vi "Boiler Controller.vi"(8 "error in":errorcluster, 9 "Controller Configuration":T1, 10 "Notifiers":T2, 11 "Message Queues":T3) -> (0 "error out":errorcluster)   [LabVIEW 2014, in "Controller.lvlib"]
uses:
  Controller.lvlib
  support/Message Queue/All Message Queues.ctl
  support/Message Queue/Message Cluster.ctl
  support/Notifiers/Notifiers.ctl
  Controller Configuration.ctl
  controls/MHL UI Data.ctl
  controls/MHL Status.ctl
  support/Boiler System Globals.vi
  <vilib>/Utility/error.llb/Error Cluster From Error Code.vi
  <vilib>/ErrorRing/Error Ring.xnode
  support/Message Queue/Message Queue.lvlib
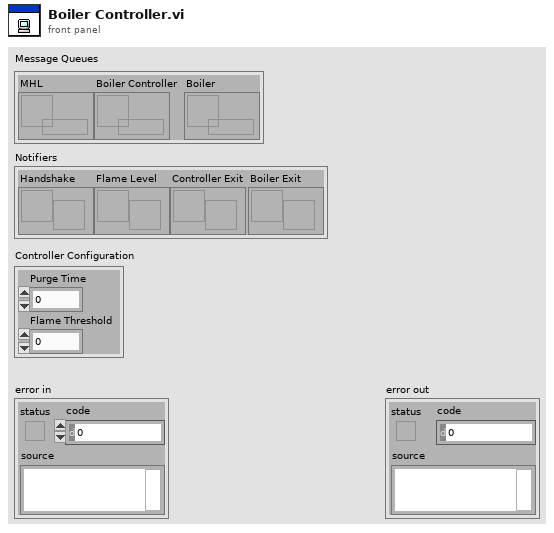
[diagram p1: front panel]
types:
  T1 = typedef "Controller.lvlib/Controller Configuration.ctl" = cluster{"Purge Time":u32, "Flame Threshold":u32}
  T2 = typedef "Notifiers.ctl" = cluster{"Handshake":refnum<notifier>, "Flame Level":refnum<notifier>, "Controller Exit":refnum<notifier>, "Boiler Exit":refnum<notifier>}
  T3 = typedef "Message Queue.lvlib/All Message Queues.ctl" = cluster{"MHL":refnum<queue>, "Boiler Controller":refnum<queue>, "Boiler":refnum<queue>}
  T4 = enum16{"open", "replace", "create", "open or create", "replace or create", "replace or create with confirmation"}
  T5 = typedef "MHL Status.ctl" = enum16{"Lockout", "Ready", "Pre-Purge", "Pre-Purge Complete", "Pilot On", "Boiler Running", "Shutdown", "Purge"}
  T6 = typedef "MHL UI Data.ctl" = cluster{"Status":string, "Fuel Control Valve":u32, "Primary Fan":bool, "Pilot Gas Valve":bool, "Pilot":bool, "Forced Draft Fan":bool, "MHL Status":T5}
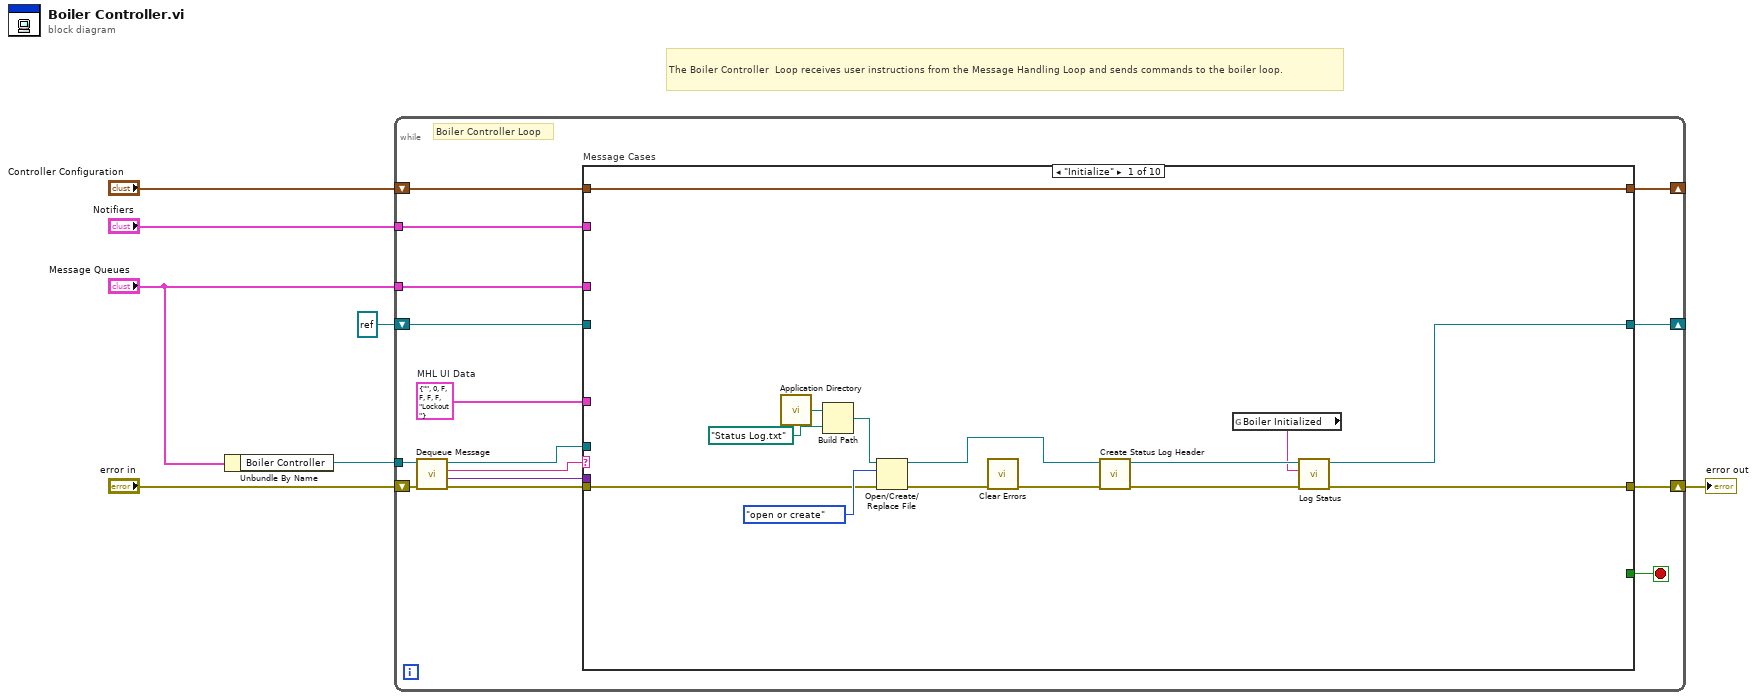
[diagram p0: block diagram]
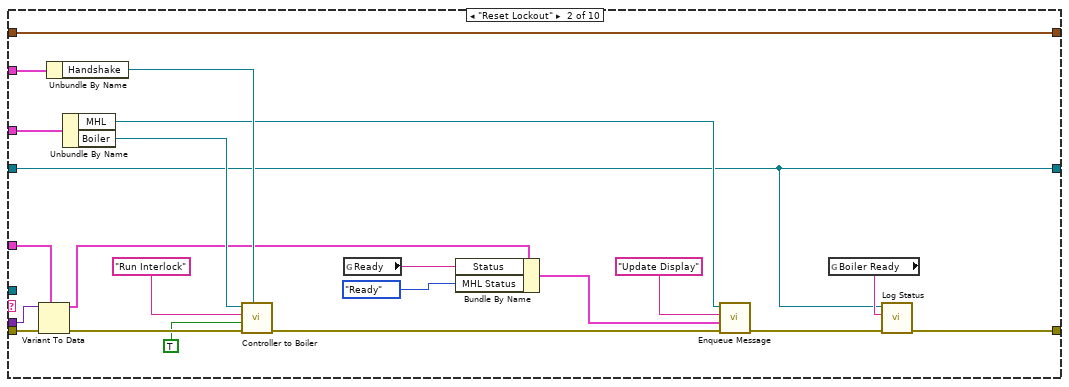
[diagram p2: hidden frame]
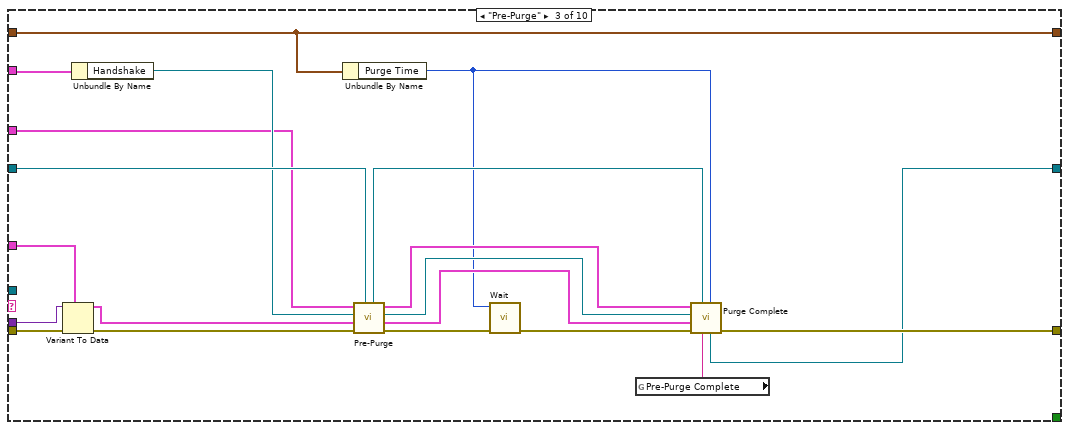
[diagram p3: hidden frame]
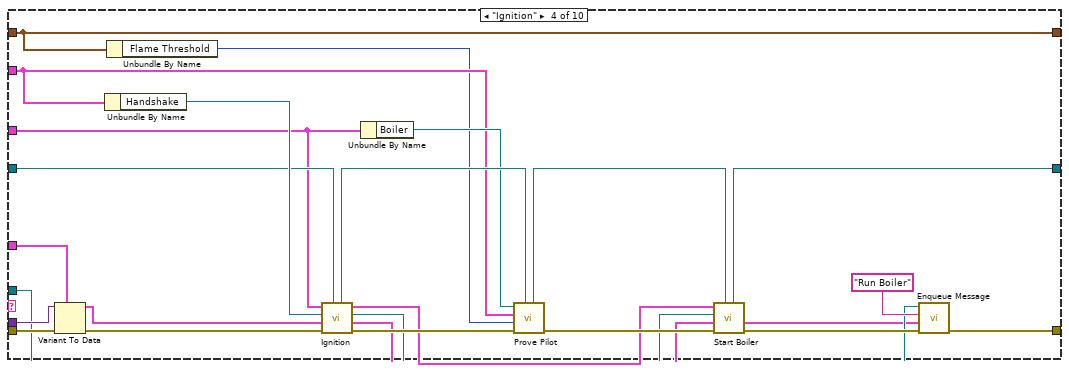
[diagram p4: hidden frame]
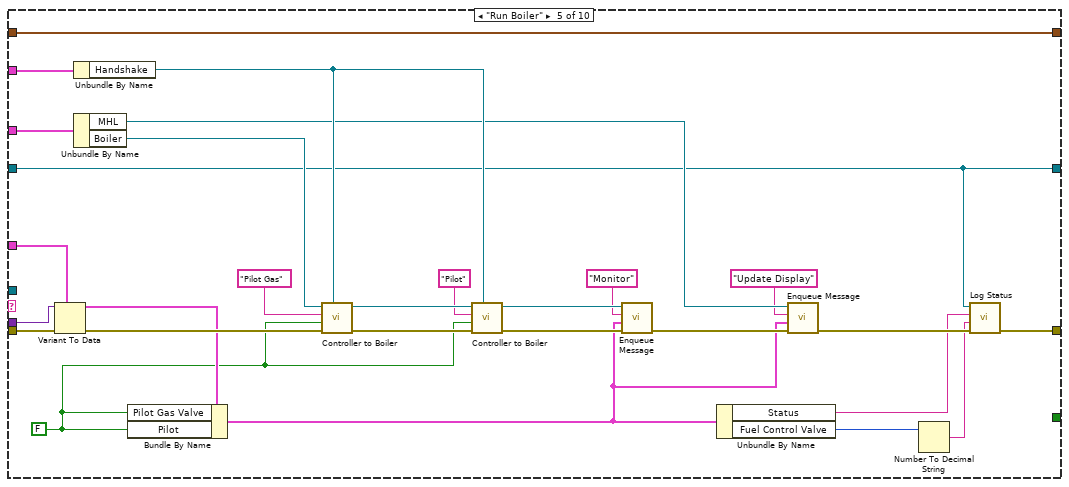
[diagram p5: hidden frame]
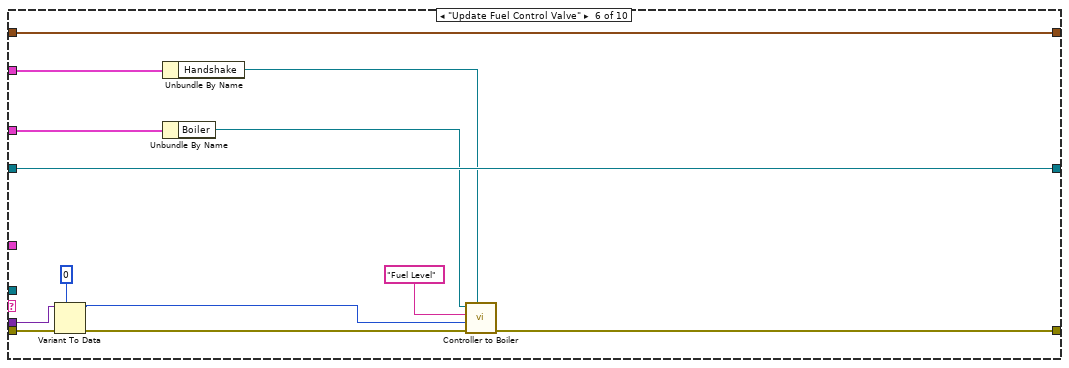
[diagram p6: hidden frame]
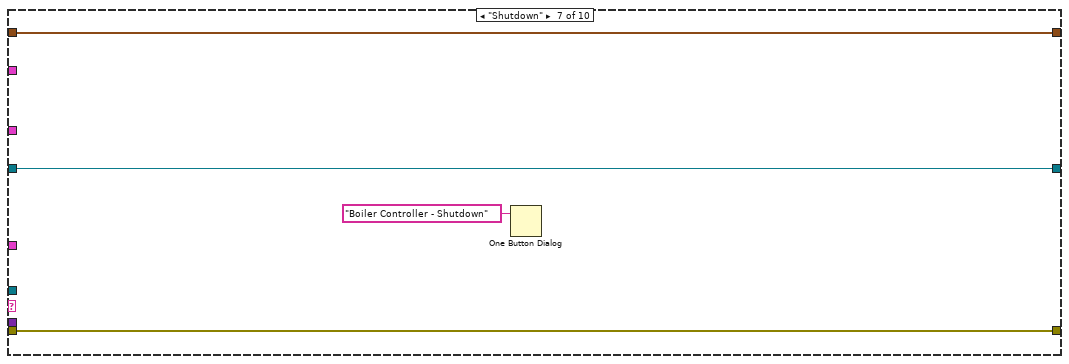
[diagram p7: hidden frame]
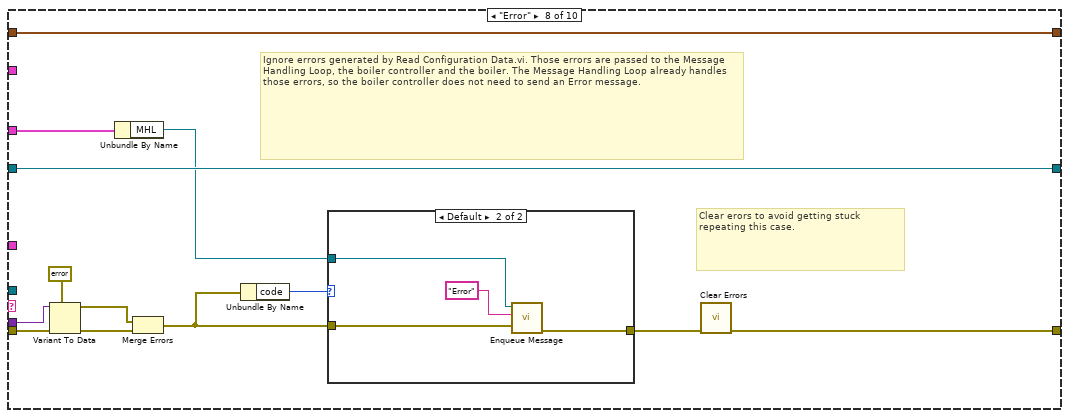
[diagram p8: hidden frame]
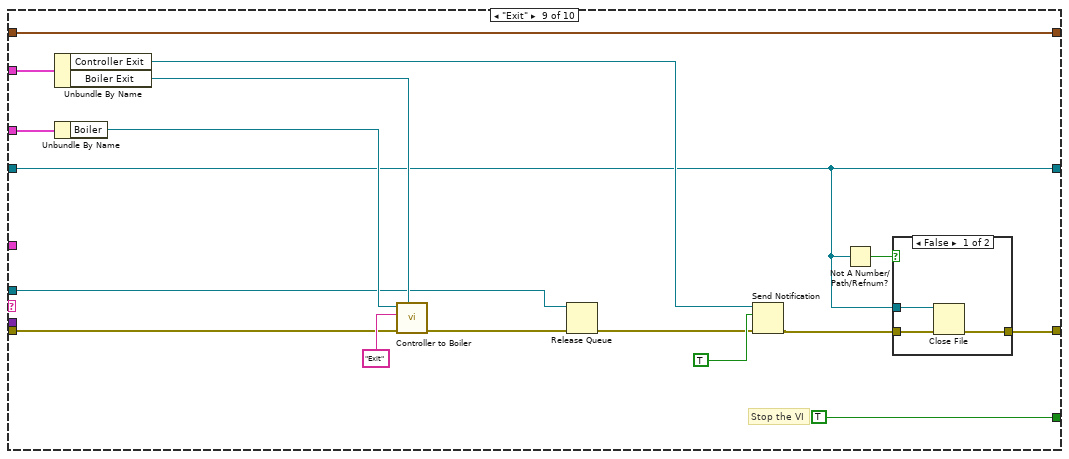
[diagram p10: hidden frame]
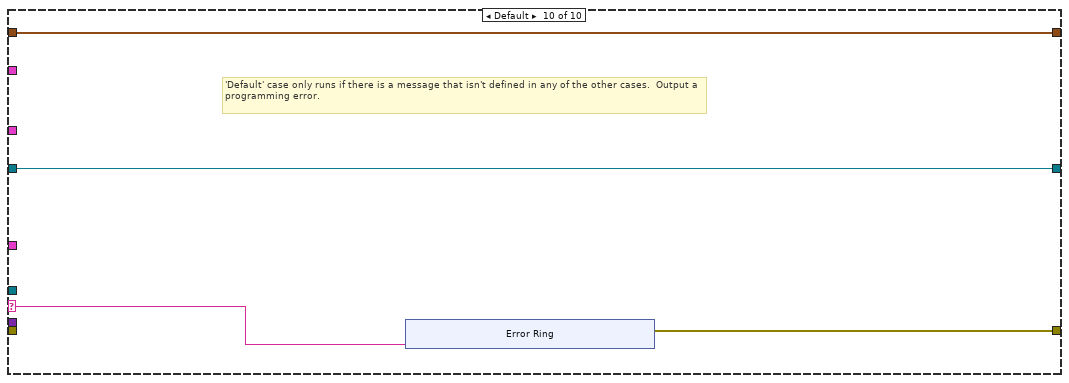
[diagram p12: hidden frame]
diagram:
  # "The Boiler Controller  Loop receives user instructions from the Message Handling Loop and sends commands to the boiler loop."
  n1 = Unbundle By Name("Message Queues") -> ("Boiler Controller"=w5:refnum<queue>)
  n2 = while {
    tunnel: w5 -> [w16]
    shift-right: [w15] -> w7
    shift-left: "error in" -> [w21]
    tunnel: "Message Queues" -> [w14]
    tunnel: "Notifiers" -> [w13]
    shift-right: [w12] -> _
    shift-left: refnum<file> refnum ("Log File Refnum out") -> [w11]
    shift-right: [w8] -> _
    shift-left: "Controller Configuration" -> [w9]
    stop <- w22 stop-if-true
    w10 = T6 {"Status"="", "Fuel Control Valve"=0, "Primary Fan"=FALSE, "Pilot Gas Valve"=FALSE, "Pilot"=FALSE, "Forced Draft Fan"=FALSE, "MHL Status"=enum."Lockout"}  # MHL UI Data
    # "Boiler Controller Loop"
    n3 = call "Dequeue Message.vi"("error in (no error)"=w21, "Message Queue"=w16) -> ("error out"=w20:errorcluster, "Message Data"=w18:variant, "Message"=w19:string, "dup Message Queue"=w17:refnum<queue>)  [unwired: 6 in]
    n4 = case "Message Cases" shown="\"Initialize\"" w19 {
      selector: w19 -> [_ _ _ _ _ _ _ _ _ w190]
      tunnel: w17 -> [_ _ _ w91 _ _ _ _ w176 _]
      tunnel: w20 -> [w26 w58 w78 w103 w131 w144 w148 w160 w175 _]
      tunnel: [w27 w54 w66 w98 w127 w140 w148 w151 w168 w191] -> w15
      tunnel: [_ _ _ _ _ _ _ _ TRUE _] -> w22
      tunnel: w18 -> [_ w53 w76 w97 w126 w139 _ w158 _ _]
      tunnel: w14 -> [_ w51 w70 w88 w122 w136 _ w161 w173 _]
      tunnel: w13 -> [_ w49 w73 w86 w121 w135 _ _ w172 _]
      tunnel: [w25 w39 w64 w79 w108 w143 w146 w155 w167 w189] -> w12
      tunnel: w11 -> [_ w39 w72 w93 w108 w143 w146 w155 w167 w189]
      tunnel: w10 -> [_ w52 w75 w96 w115 _ _ _ _ _]
      tunnel: w9 -> [w24 w37 w68 w85 w130 w142 w145 w154 w171 w188]
      tunnel: [w24 w37 w68 w85 w130 w142 w145 w154 w171 w188] -> w8
      frame "Initialize" {
        n5 = call <vilib>:"Application Directory.vi"() -> ("Application Directory"=w29:path)
        n6 = Build Path(base path=w29, name or relative path=path "Status Log.txt") -> (appended path=w33:path)
        n7 = Open/Create/Replace File(file path (use dialog)=w33, error in=w26, operation (0:open)=T4."open or create") -> (refnum out=w30:refnum<file>, error out=w31:errorcluster)  [unwired: 3 in, 1 out]
        n8 = call <vilib>:"Clear Errors.vi"("error in (no error)"=w31) -> ("error out"=w23:errorcluster)  [unwired: 5 in, 1 out]
        n9 = call "Create Status Log Header.vi"("error in"=w23, "Log File Refnum in"=w30) -> ("error out"=w36:errorcluster, "Log File Refnum out"=w35:refnum<file>)  [unwired: 8 in]
        n10 = global read "Boiler System Globals.vi" "Boiler Initialized"() -> (w34:string)
        n11 = call "Log Status.vi"("error in"=w36, "Event String"=w34, "Log File Refnum In"=w35) -> ("error out"=w27:errorcluster, "Log File Refnum Out"=w25:refnum<file>)  [unwired: 7 in]
      }
      frame "Reset Lockout" {
        n12 = Variant To Data(error in=w58, type=w52, Variant=w53) -> (data=w45:T6, error out=w57:errorcluster)
        n13 = Unbundle By Name(w49) -> ("Handshake"=w48:refnum<notifier>)
        n14 = Unbundle By Name(w51) -> ("MHL"=w41:refnum<queue>, "Boiler"=w50:refnum<queue>)
        n15 = call "Controller to Boiler.vi"("Notifier"=w48, "error in"=w57, "Message Data"=TRUE, "Message"="Run Interlock", "Boiler Queue in"=w50) -> ("error out"=w56:errorcluster)  [unwired: 4 in, 2 out]
        n16 = global read "Boiler System Globals.vi" "Ready"() -> (w44:string)
        n17 = Bundle By Name(cluster=w45, "Status"=w44, "MHL Status"=MHL_Status."Ready") -> (w43:T6)
        n18 = call "Enqueue Message.vi"("error in (no error)"=w56, "Message Data"=w43, "Message"="Update Display", "Message Queue"=w41) -> ("error out"=w55:errorcluster)  [unwired: 6 in, 1 out]
        n19 = global read "Boiler System Globals.vi" "Boiler Ready"() -> (w40:string)
        n20 = call "Log Status.vi"("error in"=w55, "Event String"=w40, "Log File Refnum In"=w39) -> ("error out"=w54:errorcluster)  [unwired: 7 in, 1 out]
      }
      frame "Pre-Purge" {
        n21 = Variant To Data(error in=w78, type=w75, Variant=w76) -> (data=w74:T6, error out=w77:errorcluster)
        n22 = Unbundle By Name(w73) -> ("Handshake"=w71:refnum<notifier>)
        n23 = Unbundle By Name(w68) -> ("Purge Time"=w60:u32)
        n24 = call "Pre-Purge.vi"("Log File Refnum in"=w72, "error in"=w77, "UI Data in"=w74, "Handshake Notifier in"=w71, "Message Queues in"=w70) -> ("error out"=w69:errorcluster, "UI Data out"=w63:T6, "Handshake Notifier out"=w62:refnum<notifier>, "Message Queues out"=w61:T3, "Log File Refnum out"=w65:refnum<file>)  [unwired: 2 in]
        n25 = call "Wait.vi"("error in"=w69, "Purge Time (s)"=w60) -> ("error out"=w67:errorcluster)  [unwired: 9 in]
        n26 = global read "Boiler System Globals.vi" "Pre-Purge Complete"() -> (w59:string)
        n27 = call "Purge Complete.vi"("Purge Time"=w60, "Status"=w59, "Log File Refnum in"=w65, "error in"=w67, "UI Data in"=w63, "Handshake Notifier in"=w62, "Message Queues in"=w61) -> ("error out"=w66:errorcluster, "Log File Refnum out"=w64:refnum<file>)  [unwired: 3 out]
      }
      frame "Ignition" {
        n28 = Variant To Data(error in=w103, type=w96, Variant=w97) -> (data=w95:T6, error out=w102:errorcluster)
        n29 = Unbundle By Name(w86) -> ("Handshake"=w94:refnum<notifier>)
        n30 = Unbundle By Name(w85) -> ("Flame Threshold"=w84:u32)
        n31 = call "Ignition.vi"("Log File Refnum in"=w93, "error in"=w102, "UI Data in"=w95, "Handshake Notifier in"=w94, "Message Queues in"=w88) -> ("error out"=w101:errorcluster, "UI Data out"=w83:T6, "Handshake Notifier out"=w82:refnum<notifier>, "Message Queues out"=w81:T3, "Log File Refnum out"=w89:refnum<file>)  [unwired: 2 in]
        n32 = Unbundle By Name(w88) -> ("Boiler"=w87:refnum<queue>)
        n33 = call "Prove Pilot.vi"("Log File Refnum in"=w89, "error in"=w101, "Flame Threshold"=w84, "Notifiers in"=w86, "Boiler Queue in"=w87) -> ("error out"=w100:errorcluster, "Log File Refnum out"=w80:refnum<file>)  [unwired: 3 in, 2 out]
        n34 = call "Start Boiler.vi"("Log File Refnum in"=w80, "error in"=w100, "UI Data in"=w83, "Handshake Notifier in"=w82, "Message Queues in"=w81) -> ("error out"=w99:errorcluster, "UI Data out"=w90:T6, "Log File Refnum out"=w79:refnum<file>)  [unwired: 2 in, 2 out]
        n35 = call "Enqueue Message.vi"("error in (no error)"=w99, "Message Data"=w90, "Message"="Run Boiler", "Message Queue"=w91) -> ("error out"=w98:errorcluster)  [unwired: 6 in, 1 out]
      }
      frame "Run Boiler" {
        w111 = FALSE ("Pilot Gas Valve")
        n36 = Variant To Data(error in=w131, type=w115, Variant=w126) -> (data=w114:T6, error out=w129:errorcluster)
        n37 = Unbundle By Name(w121) -> ("Handshake"=w120:refnum<notifier>)
        n38 = Unbundle By Name(w122) -> ("MHL"=w116:refnum<queue>, "Boiler"=w119:refnum<queue>)
        n39 = Bundle By Name(cluster=w114, "Pilot Gas Valve"=w111, "Pilot"=w111) -> (w107:T6)
        n40 = call "Controller to Boiler.vi"("Notifier"=w120, "error in"=w129, "Message Data"=w111, "Message"="Pilot Gas", "Boiler Queue in"=w119) -> ("error out"=w125:errorcluster, "Queue out"=w118:refnum<queue>)  [unwired: 4 in, 1 out]
        n41 = call "Controller to Boiler.vi"("Notifier"=w120, "error in"=w125, "Message Data"=w111, "Message"="Pilot", "Boiler Queue in"=w118) -> ("error out"=w124:errorcluster, "Queue out"=w117:refnum<queue>)  [unwired: 4 in, 1 out]
        n42 = call "Enqueue Message.vi"("error in (no error)"=w124, "Message Data"=w107, "Message"="Monitor", "Message Queue"=w117) -> ("error out"=w123:errorcluster)  [unwired: 6 in, 1 out]
        n43 = Unbundle By Name(w107) -> ("Status"=w104:string, "Fuel Control Valve"=w106:u32)
        n44 = call "Enqueue Message.vi"("error in (no error)"=w123, "Message Data"=w107, "Message"="Update Display", "Message Queue"=w116) -> ("error out"=w128:errorcluster)  [unwired: 6 in, 1 out]
        n45 = Number To Decimal String(number=w106) -> (decimal integer string=w105:string)  [unwired: 1 in]
        n46 = call "Log Status.vi"("error in"=w128, "Event Data String (-)"=w105, "Event String"=w104, "Log File Refnum In"=w108) -> ("error out"=w127:errorcluster)  [unwired: 6 in, 1 out]
      }
      frame "Update Fuel Control Valve" {
        n47 = Variant To Data(error in=w144, type=u32 0, Variant=w139) -> (data=w133:u32, error out=w141:errorcluster)
        n48 = Unbundle By Name(w135) -> ("Handshake"=w134:refnum<notifier>)
        n49 = Unbundle By Name(w136) -> ("Boiler"=w137:refnum<queue>)
        n50 = call "Controller to Boiler.vi"("Notifier"=w134, "error in"=w141, "Message Data"=w133, "Message"="Fuel Level", "Boiler Queue in"=w137) -> ("error out"=w140:errorcluster)  [unwired: 4 in, 2 out]
      }
      frame "Shutdown" {
        n51 = One Button Dialog(message="Boiler Controller - Shutdown") -> ()  [unwired: 1 in, 1 out]
      }
      frame "Error" {
        # "Ignore errors generated by Read Configuration Data.vi. Those errors are passed to the Message Handling Loop, the boiler controller and the boiler. The Message Handling Loop already handles those errors, so the boiler controller does not need to send an Error message."
        # "Clear erors to avoid getting stuck repeating this case."
        n52 = Variant To Data(error in=w160, type=errorcluster {"status"=FALSE, "code"=0, "source"=""} ("error out"), Variant=w158) -> (data=w156:errorcluster, error out=w157:errorcluster)
        n53 = Unbundle By Name(w161) -> ("MHL"=w150:refnum<queue>)
        n54 = Merge Errors(w156, w157) -> (w149:errorcluster)
        n55 = Unbundle By Name(w149) -> ("code"=w152:i32)
        n56 = case shown="Default" w152 {
          tunnel: w150 -> [_ w165]
          tunnel: [w162 w164] -> w153
          tunnel: w149 -> [w162 w163]
          frame 5000..5002 {
          }
          frame Default {
            n57 = call "Enqueue Message.vi"("Message Data"=w163, "Message"="Error", "Message Queue"=w165) -> ("error out"=w164:errorcluster)  [unwired: 7 in, 1 out]
          }
        }
        n58 = call <vilib>:"Clear Errors.vi"("error in (no error)"=w153) -> ("error out"=w151:errorcluster)  [unwired: 5 in, 1 out]
      }
      frame "Exit" {
        # "Stop the VI"
        n59 = Unbundle By Name(w172) -> ("Controller Exit"=w178:refnum<notifier>, "Boiler Exit"=w180:refnum<notifier>)
        n60 = Unbundle By Name(w173) -> ("Boiler"=w177:refnum<queue>)
        n61 = call "Controller to Boiler.vi"("Notifier"=w180, "error in"=w175, "Message"="Exit", "Boiler Queue in"=w177) -> ("error out"=w183:errorcluster)  [unwired: 5 in, 2 out]
        n62 = Release Queue(queue=w176, error in (no error)=w183) -> (error out=w179:errorcluster)  [unwired: 1 in, 2 out]
        n63 = Send Notification(notification=TRUE, notifier=w178, error in (no error)=w179) -> (error out=w169:errorcluster)  [unwired: 1 out]
        n64 = Not A Number/Path/Refnum?(number/path/refnum=w167) -> (NaN/Path/Refnum?=w170:bool)
        n65 = case shown="False" w170 {
          tunnel: [w185 w187] -> w168
          tunnel: w169 -> [w186 w187]
          tunnel: w167 -> [w184 _]
          frame False {
            n66 = Close File(refnum=w184, error in=w186) -> (error out=w185:errorcluster)  [unwired: 1 out]
          }
          frame True {
          }
        }
      }
      frame Default {
        # "'Default' case only runs if there is a message that isn't defined in any of the other cases.  Output a programming error."
        n67 = xnode "Error Ring"("parameter 0"=w190) -> ("error out"=w191:errorcluster)
      }
    }
  }
  "error out" <- w7
